vi "total_valve_control.vi"() -> ()   [LabVIEW 2014]
panel:
  in  "Read Pirani pressure?":bool
  in  "Read CC pressure?":bool
  out "Valve 2 Closed?":bool
  out "Valve 1 Closed?":bool
  out "Valve 3 Closed?":bool
  out "Cold Cathode Gauge Pressure [Torr]":dbl
  out "Valve Percentage Open":dbl
  out "Unacceptable Flow Rate Value":bool
  in  "Enter Flow Rate (mbar*Liters/sec)":dbl
  out "Pirani Gauge Pressure [Torr]":dbl
  out "Valve 2 Open?":bool
  out "Valve 2, value 2":dbl format="%0.2f"
  out "Valve 2, value 1":dbl format="%0.2f"
  out "Valve 1, value 2":dbl format="%0.2f"
  out "Valve 1, value 1":dbl format="%0.2f"
  out "Valve 3, value 2":dbl format="%0.2f"
  out "Valve 3, value 1":dbl format="%0.2f"
  in  "?":bool
  out "Valve 3 Open?":bool
  out "Valve 1 Open?":bool
  in  "Open Valve 2?":bool
  in  "Open Valve 3?":bool
  in  "Open Valve 1?":bool
  # "ROUGHING\nPUMP"
  # "Valve 1"
  # "Valve 3"
  # "TURBO"
  # "Valve 2"
  # "Vent Valve"
  # "CHAMBER"
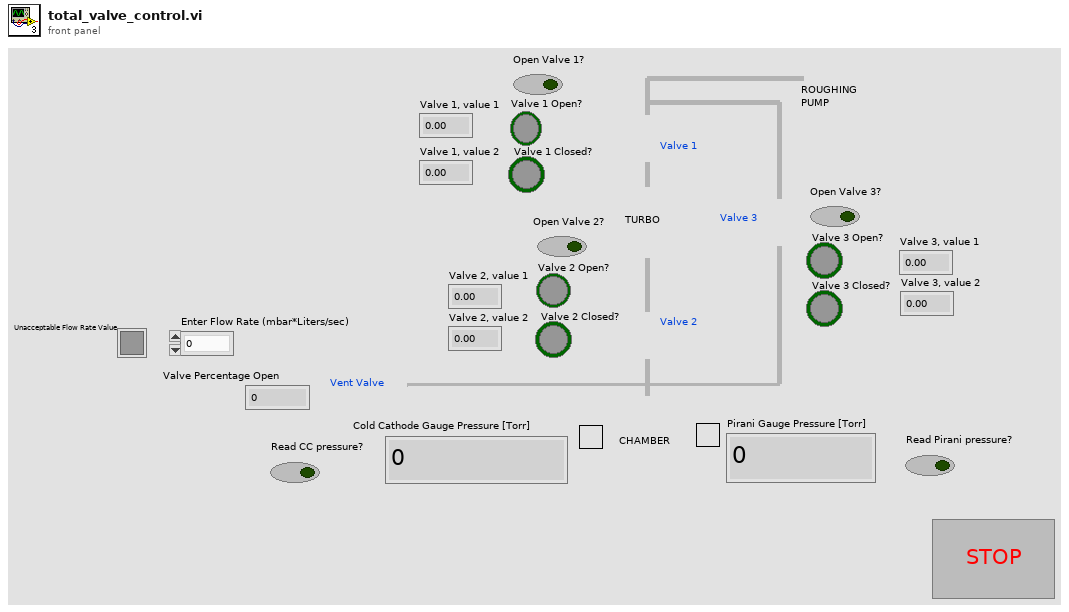
[diagram p1: front panel]
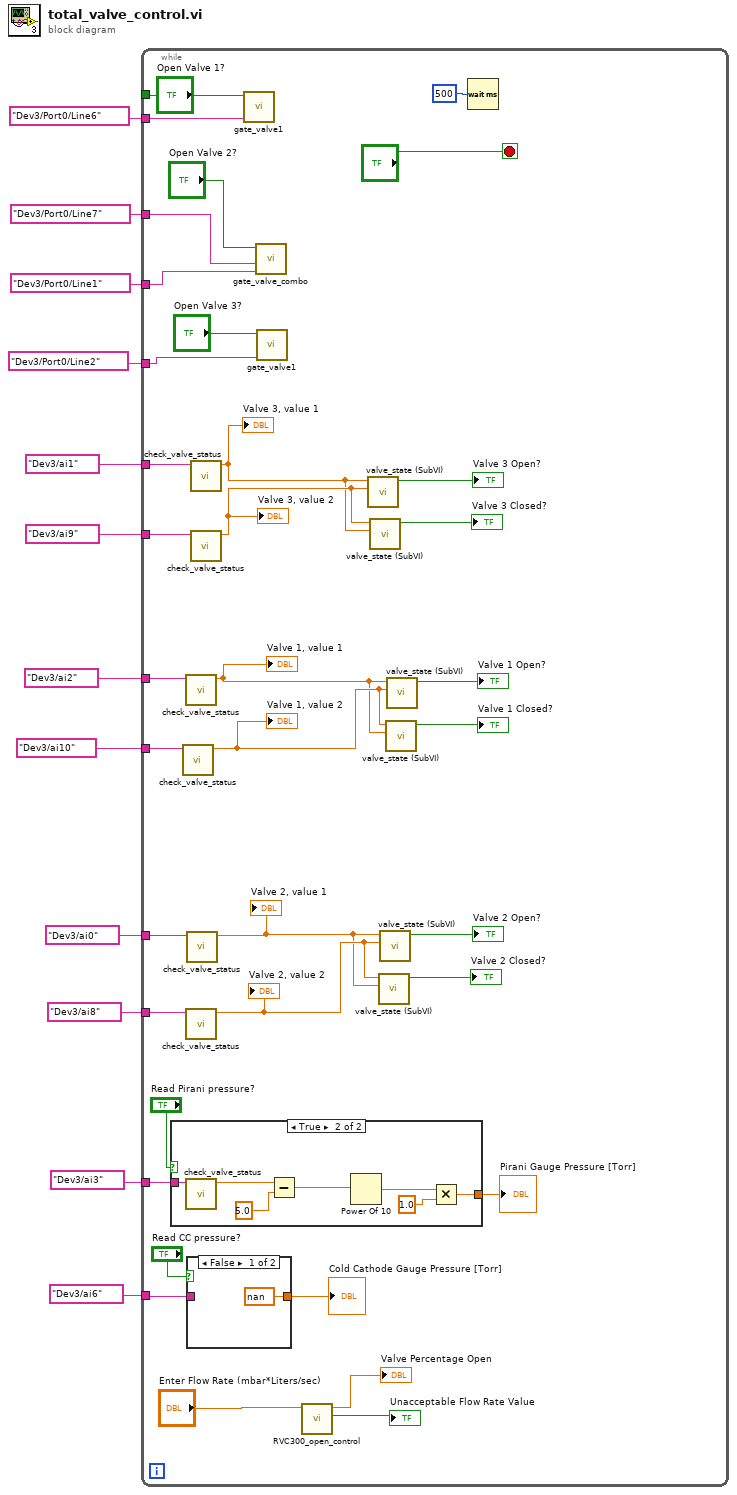
[diagram p0: block diagram]
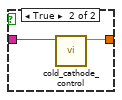
[diagram p2: hidden frame]
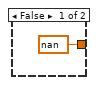
[diagram p3: hidden frame]
diagram:
  n1 = while {
    tunnel: tag "Dev3/ai2" ("Valve 1 Ch. 1") -> [w48]
    tunnel: tag "Dev3/ai10" ("Valve 1 Ch. 2") -> [w47]
    tunnel: tag "Dev3/ai1" ("Valve 3 Ch. 1") -> [w46]
    tunnel: tag "Dev3/ai9" ("Valve 3 Ch. 2") -> [w45]
    tunnel: ["Open Valve 1?"] -> _
    tunnel: tag "Dev3/Port0/Line6" ("Control Valve 1") -> [w43]
    tunnel: tag "Dev3/Port0/Line2" ("Control Valve  3") -> [w40]
    tunnel: tag "Dev3/Port0/Line7" ("Control Valve 2") -> [w41]
    tunnel: tag "Dev3/Port0/Line1" ("Channel for Valve Pair 2") -> [w42]
    tunnel: tag "Dev3/ai0" ("Channel 1") -> [w34]
    tunnel: tag "Dev3/ai8" ("Channel 1") -> [w33]
    tunnel: tag "Dev3/ai3" ("Channel 1") -> [w32]
    tunnel: tag "Dev3/ai6" ("Cold Cathode Gauge Channel") -> [w27]
    stop <- "?" stop-if-true
    n2 = case shown="True" "Read Pirani pressure?" {
      tunnel: w32 -> [_ w59]
      tunnel: [nan w53] -> w31
      frame False {
      }
      frame True {
        n3 = call "check_valve_status.vi"("Channel 1"=w59) -> ("Ch. 1 value"=w57:dbl)  [unwired: 10 in]
        n4 = Subtract(x=w57, y=5.0) -> (x-y=w56:dbl)
        n5 = Power Of 10(x=w56) -> (10^x=w55:dbl)
        n6 = Multiply(x=w55, y=1.0) -> (x*y=w53:dbl)
      }
    }
    "Pirani Gauge Pressure [Torr]" <- w31
    n7 = call "check_valve_status.vi"("Channel 1"=w47) -> ("Ch. 1 value"=w21:dbl)  [unwired: 10 in]
    "Valve 1, value 2" <- w21
    n8 = call "check_valve_status.vi"("Channel 1"=w48) -> ("Ch. 1 value"=w20:dbl)  [unwired: 10 in]
    "Valve 1, value 1" <- w20
    n9 = call "check_valve_status.vi"("Channel 1"=w33) -> ("Ch. 1 value"=w18:dbl)  [unwired: 10 in]
    "Valve 2, value 2" <- w18
    n10 = call "check_valve_status.vi"("Channel 1"=w34) -> ("Ch. 1 value"=w17:dbl)  [unwired: 10 in]
    "Valve 2, value 1" <- w17
    n11 = case shown="False" "Read CC pressure?" {
      tunnel: w27 -> [_ w51]
      tunnel: [nan ("Cold Cathode Gauge Pressure") w50] -> w26
      frame False {
      }
      frame True {
        n12 = call "cold_cathode_control.vi"("Cold Cathode Gauge Channel"=w51) -> ("Cold Cathode Gauge Pressure"=w50:dbl)  [unwired: 10 in]
      }
    }
    "Cold Cathode Gauge Pressure [Torr]" <- w26
    n13 = call "check_valve_status.vi"("Channel 1"=w46) -> ("Ch. 1 value"=w24:dbl)  [unwired: 10 in]
    "Valve 3, value 1" <- w24
    n14 = call "check_valve_status.vi"("Channel 1"=w45) -> ("Ch. 1 value"=w25:dbl)  [unwired: 10 in]
    "Valve 3, value 2" <- w25
    n15 = call "gate_valve1.vi"("Open Valve?"="Open Valve 1?", "physical channels"=w43) -> ()  [unwired: 9 in]
    n16 = call "gate_valve_combo.vi"("Channel for Valve Pair 2"=w42, "Channel for Valve Pair 1"=w41, "Open Gate Valve?"="Open Valve 2?") -> ()  [unwired: 9 in]
    n17 = call "gate_valve1.vi"("Open Valve?"="Open Valve 3?", "physical channels"=w40) -> ()  [unwired: 9 in]
    n18 = call "RVC300_open_control.vi"("Enter Flow Rate (mbar*Liters/sec)"="Enter Flow Rate (mbar*Liters/sec)") -> ("Unacceptable Flow Rate Value"=→"Unacceptable Flow Rate Value":bool, "Valve Percentage Open"=→"Valve Percentage Open":dbl)  [unwired: 9 in]
    n19 = call "valve_state (SubVI).vi"("Ch. 1 value 2"=w25, "Ch. 1 value"=w24) -> ("Boolean"=→"Valve 3 Open?":bool)  [unwired: 9 in]
    n20 = call "valve_state (SubVI).vi"("Ch. 1 value 2"=w24, "Ch. 1 value"=w25) -> ("Boolean"=→"Valve 3 Closed?":bool)  [unwired: 9 in]
    n21 = call "valve_state (SubVI).vi"("Ch. 1 value 2"=w17, "Ch. 1 value"=w18) -> ("Boolean"=→"Valve 2 Closed?":bool)  [unwired: 9 in]
    n22 = call "valve_state (SubVI).vi"("Ch. 1 value 2"=w18, "Ch. 1 value"=w17) -> ("Boolean"=→"Valve 2 Open?":bool)  [unwired: 9 in]
    n23 = call "valve_state (SubVI).vi"("Ch. 1 value 2"=w20, "Ch. 1 value"=w21) -> ("Boolean"=→"Valve 1 Closed?":bool)  [unwired: 9 in]
    n24 = call "valve_state (SubVI).vi"("Ch. 1 value 2"=w21, "Ch. 1 value"=w20) -> ("Boolean"=→"Valve 1 Open?":bool)  [unwired: 9 in]
    n25 = Wait (ms)(milliseconds to wait=u32 500) -> ()  [unwired: 1 out]
  }
